vi "将启用的浓度作为新的浓度数组.vi"(0 "启用布尔数组":bool[](array[boolean]), 5 "输入浓度数组":dbl[](array[numeric])) -> (4 "启用的浓度数组":dbl[](array[numeric]))   [LabVIEW 2016, in "斯坦道CODMn.lvlib"]
panel:
  in  "启用5":bool
  in  "启用4":bool
  in  "启用3":bool
  in  "启用2":bool
  in  "启用1":bool
  in  "浓度5":dbl
  in  "浓度4":dbl
  in  "浓度3":dbl
  in  "浓度2":dbl
  in  "浓度1":dbl
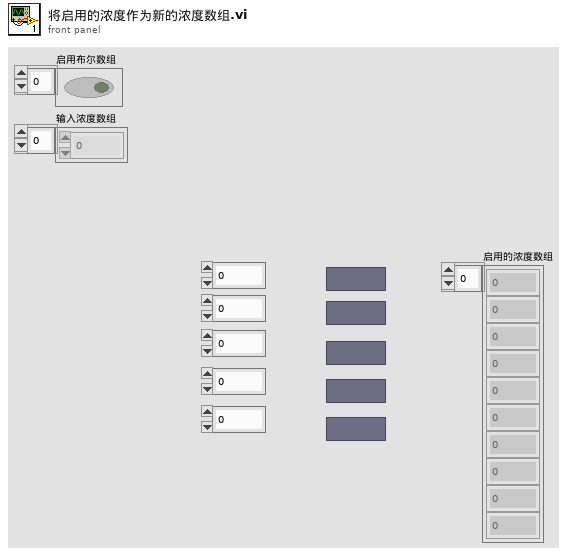
[diagram p1: front panel]
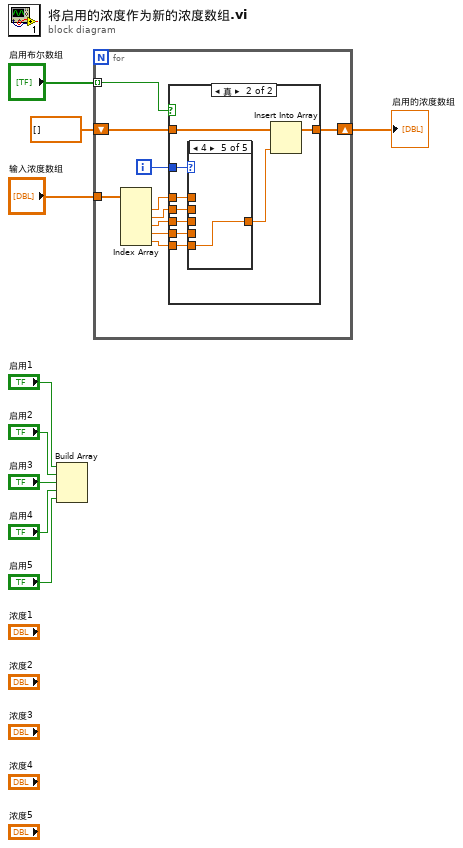
[diagram p0: block diagram]
diagram:
  n1 = Build Array("启用1", "启用2", "启用3", "启用4", "启用5") -> ()  [unwired: 1 out]
  n2 = for {
    tunnel: "启用布尔数组" -> [w19] mode=indexing
    shift-right: [w17] -> w3
    shift-left: dbl[] [] ("数组") -> [w16]
    tunnel: "输入浓度数组" -> [w15]
    i -> [w18]
    n3 = Index Array(array=w15) -> (element #1=w14:dbl, element #2=w13:dbl, element #3=w12:dbl, element #4=w11:dbl, element #5=w10:dbl)  [unwired: 5 in]
    n4 = case shown="真" w19 {
      tunnel: w18 -> [_ w29]
      tunnel: [w20 w27] -> w17
      tunnel: w16 -> [w20 w26]
      tunnel: w14 -> [_ w25]
      tunnel: w13 -> [_ w24]
      tunnel: w12 -> [_ w23]
      tunnel: w11 -> [_ w22]
      tunnel: w10 -> [_ w21]
      frame False {
      }
      frame True {
        n5 = case shown="4" w29 {
          tunnel: [w30 w31 w32 w33 w34] -> w28
          tunnel: w25 -> [w30 _ _ _ _]
          tunnel: w24 -> [_ w31 _ _ _]
          tunnel: w23 -> [_ _ w32 _ _]
          tunnel: w22 -> [_ _ _ w33 _]
          tunnel: w21 -> [_ _ _ _ w34]
          frame 0, Default {
          }
          frame 1 {
          }
          frame 2 {
          }
          frame 3 {
          }
          frame 4 {
          }
        }
        n6 = Insert Into Array(array=w26, new element=w28) -> (w27:dbl[])  [unwired: 1 in]
      }
    }
  }
  "启用的浓度数组" <- w3
